vi "ukol1.vi"() -> ()   [LabVIEW 2023]
uses:
  <vilib>/measure/maspectr.llb/FFT Spectrum (Mag-Phase) for 1 Chan.vi
  <vilib>/addons/Digital Filter Design/Process.llb/DFD Filtering (Wfm).vi
  <vilib>/addons/Digital Filter Design/Process.llb/DFD Integer Delay (Array).vi
  <vilib>/measure/NI_MABase.lvlib
  <vilib>/addons/Digital Filter Design/NI_DigFilterLicensed.lvlib
  <vilib>/measure/NI_MAPro.lvlib
panel:
  out "Waveform Graph 8":waveform(dbl)[](graph)
  out "Waveform Graph 7":waveform(dbl)[](graph)
  out "Waveform Graph 6":cluster{"f0":dbl, "df":dbl, "magnitude":dbl[]}[](graph)
  out "Waveform Graph 5":cluster{"f0":dbl, "df":dbl, "magnitude":dbl[]}[](graph)
  out "Waveform Graph 4":cluster{"f0":dbl, "df":dbl, "magnitude":dbl[]}[](graph)
  out "Waveform Graph 3":cluster{"f0":dbl, "df":dbl, "magnitude":dbl[]}[](graph)
  out "Waveform Graph 2":waveform(dbl)[](graph)
  out "Waveform Graph":waveform(dbl)[](graph)
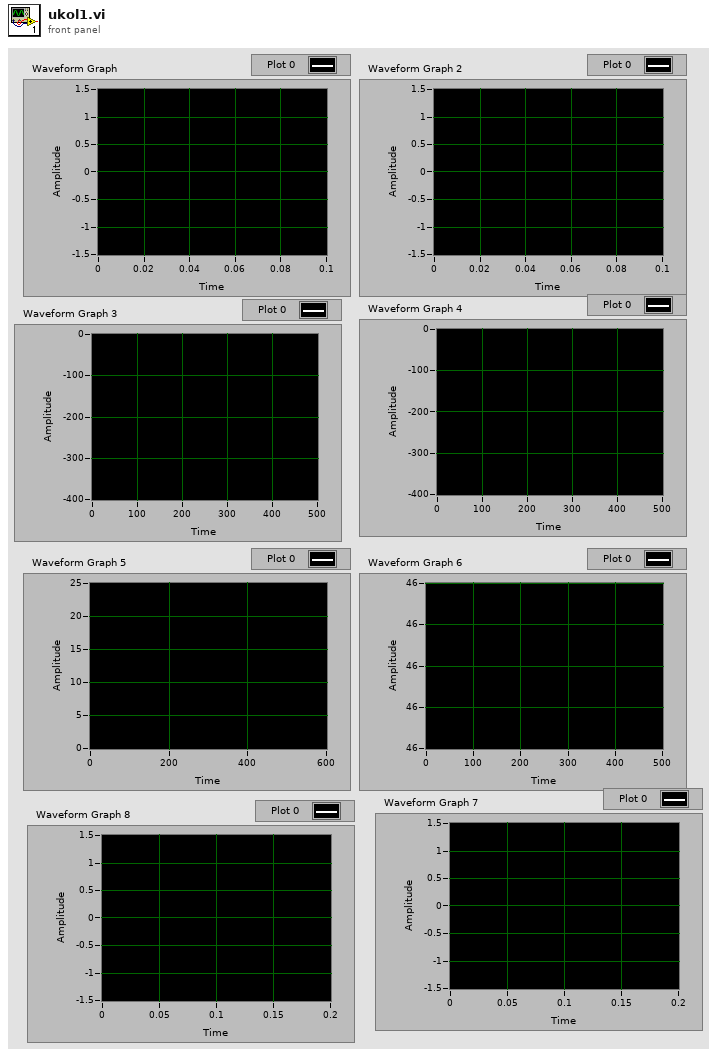
[diagram p1: front panel]
types:
  T1 = typedef "NI_DigFilterLicensed.lvlib/DFD Filter Obj.ctl" = cluster{"mSRate_Fs":dbl, "mSRate_Version":string, "mSRate_Comments":string, "mSRate_OrgCoef":T2, "mSRate_CurCoef":T2, "mSRate_Quantized?":bool, "mSRate_QCoef":T2, "mSRate_QSettings":T4[], "mSRate_Order":i32, "mSRate_Scaling":cluster{"mSRate_ScaleByPowerOf2?":bool, "mSRate_ScaleType":T6}}
  T2 = typedef "NI_DigFilterLicensed.lvlib/DFD Filter Coef.ctl" = cluster{"type":T3, "gain":dbl, "coef a (k)":dbl[], "coef b (v)":dbl[]}
  T3 = typedef "NI_DigFilterLicensed.lvlib/DFD Filter Structure Type Selector.ctl" = enum16{"Undefined", "FIR Direct Form", "FIR Direct Form Transposed", "FIR Symmetric", "FIR Antisymmetric", "IIR Direct Form I", "IIR Direct Form I Transposed", "IIR Direct Form II", "IIR Direct Form II Transposed", "IIR Cascaded Second Order Sections Form I", "IIR Cascaded Second Order Sections Form I Transposed", "IIR Cascaded Second Order Sections Form II", "IIR Cascaded Second Order Sections Form II Transposed", "Lattice Allpass (basic sections)", "Lattice Allpass (one multiplier sections)", "Lattice Allpass (normalized sections)", "Lattice AR (basic sections)", "Lattice AR (one multiplier sections)", "Lattice AR (normalized sections)", "Lattice MA (minimum phase)", "Lattice MA (maximum phase)", "Lattice ARMA (basic sections)", "Lattice ARMA (one multiplier sections)", "Lattice ARMA (normalized sections)"}
  T4 = typedef "NI_DigFilterLicensed.lvlib/dfd_Internal Quantization Settings.ctl" = cluster{"source":T5, "wl":i16, "iwl":i16, "overflow mode":enum16{"Saturation", "Wrap"}, "rounding mode":enum16{"Nearest", "Truncation"}, "signed?":bool}
  T5 = typedef "NI_DigFilterLicensed.lvlib/dfd_Internal Quantization Srcs.ctl" = u16
  T6 = typedef "NI_DigFilterLicensed.lvlib/DFD Coef Norm Type.ctl" = enum16{"No Norm", "Time Domain 1-Norm", "Time Domain 2-Norm", "Time Domain Inf-Norm"}
  T7 = cluster{"dB On (F)":bool, "unwrap phase (F)":bool, "convert to degree (F)":bool}
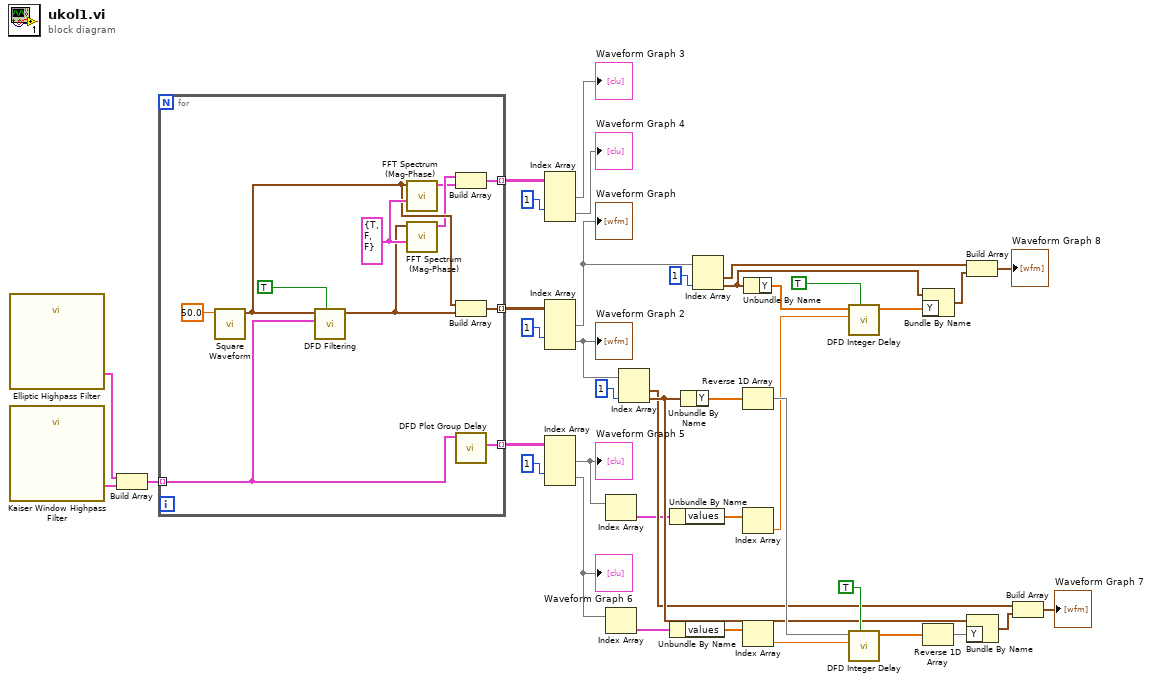
[diagram p0: block diagram]
diagram:
  n1 = call "Elliptic Highpass Filter"() -> ("filter out"=w39:T1)  [unwired: 10 in, 1 out]
  n2 = call "Kaiser Window Highpass Filter"() -> ("filter out"=w38:T1)  [unwired: 10 in, 1 out]
  n3 = Build Array(w39, w38) -> (w37:T1[])
  n4 = for {
    tunnel: w37 -> [w42] mode=indexing
    tunnel: [w46] -> w36 mode=indexing
    tunnel: [w43] -> w31 mode=indexing
    tunnel: [w41] -> w29 mode=indexing
    w48 = T7 {"dB On (F)"=TRUE, "unwrap phase (F)"=FALSE, "convert to degree (F)"=FALSE} ("view")
    n5 = call <vilib>:"Square Waveform.vi"("frequency"=50.0) -> ("signal out"=w47:waveform(dbl))  [unwired: 9 in, 1 out]
    n6 = call-poly <vilib>:"DFD Filtering.vi"("init? (F)"=TRUE, "filter"=w42, "signal in"=w47) -> ("signal out"=w40:waveform(dbl))  [unwired: 7 in, 1 out]
    n7 = call-poly <vilib>:"FFT Spectrum (Mag-Phase).vi"("view"=w48, "time signal"=w47) -> ("magnitude"=w44:cluster{"f0":dbl, "df":dbl, "magnitude":dbl[]})  [unwired: 5 in, 4 out]
    n8 = call-poly <vilib>:"FFT Spectrum (Mag-Phase).vi"("view"=w48, "time signal"=w40) -> ("magnitude"=w45:cluster{"f0":dbl, "df":dbl, "magnitude":dbl[]})  [unwired: 5 in, 4 out]
    n9 = Build Array(w45, w44) -> (w43:cluster{"f0":dbl, "df":dbl, "magnitude":dbl[]}[])
    n10 = Build Array(w47, w40) -> (w46:waveform(dbl)[])
    n11 = call <vilib>:"DFD Plot Group Delay.vi"("filter in"=w42) -> ("group delay"=w41:cluster{"f0":dbl, "df":dbl, "values":dbl[]}[])  [unwired: 8 in, 2 out]
  }
  n12 = Index Array(array=w31, index (row) #2=1 ("index (row)")) -> (element #1=→"Waveform Graph 3":cluster{"f0":dbl, "df":dbl, "magnitude":dbl[]}[], element #2=→"Waveform Graph 4":cluster{"f0":dbl, "df":dbl, "magnitude":dbl[]}[])  [unwired: 3 in]
  n13 = Index Array(array=w36, index (row) #2=1 ("index (row)")) -> (element #1=w12:waveform(dbl)[], element #2=w24:waveform(dbl)[])  [unwired: 3 in]
  "Waveform Graph" <- w12
  "Waveform Graph 2" <- w24
  n14 = Index Array(array=w29, index (row) #2=1 ("index (row)")) -> (element #1=w9:cluster{"f0":dbl, "df":dbl, "values":dbl[]}[], element #2=w28:cluster{"f0":dbl, "df":dbl, "values":dbl[]}[])  [unwired: 3 in]
  "Waveform Graph 5" <- w9
  "Waveform Graph 6" <- w28
  n15 = Index Array(array=w9) -> (element=w11:cluster{"f0":dbl, "df":dbl, "values":dbl[]})  [unwired: 1 in]
  n16 = Index Array(array=w28) -> (element=w27:cluster{"f0":dbl, "df":dbl, "values":dbl[]})  [unwired: 1 in]
  n17 = Index Array(array=w24, index #2=1 ("index")) -> (element #1=w15:waveform(dbl), element #2=w18:waveform(dbl))  [unwired: 1 in]
  n18 = Unbundle By Name(w11) -> ("values"=w10:dbl[])
  n19 = Unbundle By Name(w27) -> ("values"=w26:dbl[])
  n20 = Unbundle By Name(w18) -> ("Y"=w22:dbl[])
  n21 = Index Array(array=w12, index #2=1 ("index")) -> (element #1=w1:waveform(dbl), element #2=w4:waveform(dbl))  [unwired: 1 in]
  n22 = Reverse 1D Array(array=w22) -> (reversed array=w23:dbl[])
  n23 = Index Array(array=w10) -> (element=w6:dbl)  [unwired: 1 in]
  n24 = Index Array(array=w26) -> (element=w25:dbl)  [unwired: 1 in]
  n25 = Unbundle By Name(w4) -> ("Y"=w7:dbl[])
  n26 = call-poly <vilib>:"DFD Integer Delay.vi"("init? (F)"=TRUE, "delay"=w6, "signal in"=w7) -> ("signal out"=w5:dbl[])  [unwired: 7 in, 1 out]
  n27 = call-poly <vilib>:"DFD Integer Delay.vi"("init? (F)"=TRUE, "delay"=w25, "signal in"=w23) -> ("signal out"=w20:dbl[])  [unwired: 7 in, 1 out]
  n28 = Bundle By Name(cluster=w4, "Y"=w5) -> (w2:waveform(dbl))
  n29 = Reverse 1D Array(array=w20) -> (reversed array=w19:dbl[])
  n30 = Build Array(w1, w2) -> (→"Waveform Graph 8":waveform(dbl)[])
  n31 = Bundle By Name(cluster=w18, "Y"=w19) -> (w16:waveform(dbl))
  n32 = Build Array(w15, w16) -> (→"Waveform Graph 7":waveform(dbl)[])
